vi "Read Task Factory CMD.vi"(8 "error in (no error)":errorcluster, 11 "Task Factory MSG in":refnum<class "Task Factory MSG.lvclass">) -> (0 "error out":errorcluster, 2 "Task Factory CMD":T1 caption="Enum 3", 3 "Task Factory MSG out":refnum<class "Task Factory MSG.lvclass">)   [LabVIEW 2024, in "Task Factory MSG.lvclass"]
uses:
  Task Factory MSG.lvclass
  Type Def/Task Factory CMD.ctl
  Task Factory MSG.lvclass/Task Factory MSG.ctl
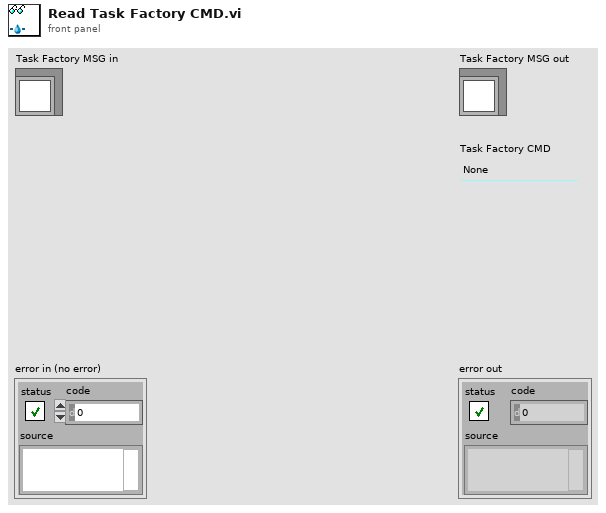
[diagram p1: front panel]
types:
  T1 = typedef "Task Factory CMD.ctl" = enum16{"None", "Generate Task"}
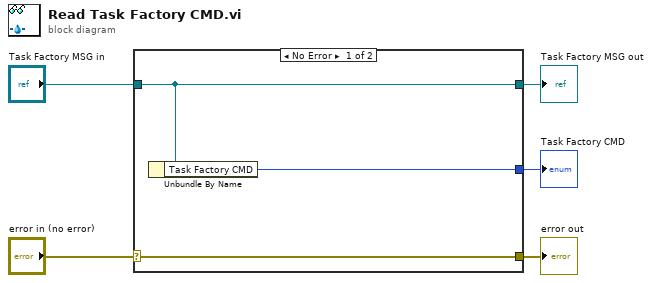
[diagram p0: block diagram]
diagram:
  n1 = case shown="No Error" "error in (no error)" {
    selector: "error in (no error)" -> [w8 w9]
    tunnel: [w8 w9] -> w4
    tunnel: [w7 w10] -> w2
    tunnel: "Task Factory MSG in" -> [w7 w10]
    tunnel: [w6 _] -> w1
    frame No Error {
      n2 = Unbundle By Name(w7) -> ("Task Factory CMD"=w6:T1)
    }
    frame Error {
    }
  }
  "error out" <- w4
  "Task Factory MSG out" <- w2
  "Task Factory CMD" <- w1
